vi "Player Info.vi"(11 "Circle the Wagons in":refnum<class "Circle the Wagons.lvclass">) -> (1 "Victory Speech":string, 2 "Name":string, 3 "Circle the Wagons out":refnum<class "Circle the Wagons.lvclass">)   [LabVIEW 2015, in "Circle the Wagons.lvclass"]
uses:
  Circle the Wagons.lvclass
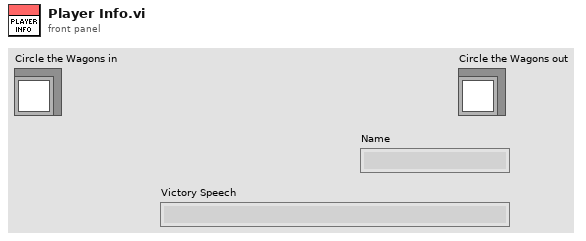
[diagram p1: front panel]
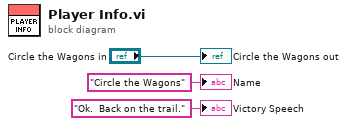
[diagram p0: block diagram]
diagram:
  "Circle the Wagons out" <- "Circle the Wagons in"
  "Name" <- "Circle the Wagons" ("Name")
  "Victory Speech" <- "Ok.  Back on the trail." ("Victory Speech")
